vi "res_REAL_offset.vi"(10 "ST_results_info":T1, 11 "REAL_position":i32) -> (3 "results_byte_array_offset":i32)   [LabVIEW 2020]
uses:
  ST_results_info.ctl
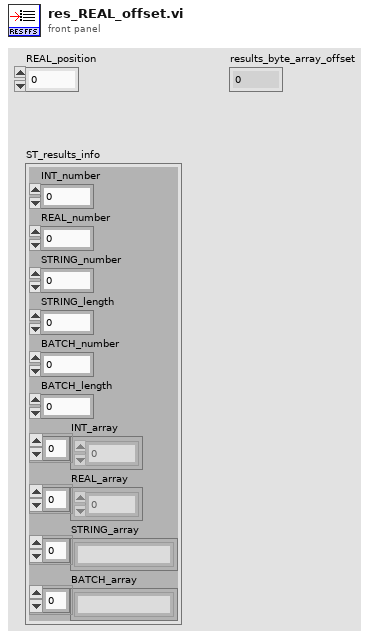
[diagram p1: front panel]
types:
  T1 = typedef "ST_results_info.ctl" = cluster{"INT_number":i32, "REAL_number":i32, "STRING_number":i32, "STRING_length":i32, "BATCH_number":i32, "BATCH_length":i32, "INT_array":i16[], "REAL_array":sgl[], "STRING_array":string[], "BATCH_array":string[]}
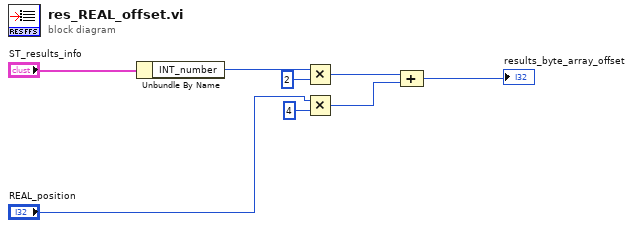
[diagram p0: block diagram]
diagram:
  n1 = Unbundle By Name("ST_results_info") -> ("INT_number"=w7:i32)
  n2 = Multiply(x=w7, y=2) -> (x*y=w4:i32)
  n3 = Multiply(x="REAL_position", y=4) -> (x*y=w3:i32)
  n4 = Compound Arithmetic op=ADD(w4, w3) -> (→"results_byte_array_offset":i32)
